vi "svc_Conditional Merge Array of Errors.vi"(7 "condition met":bool[](array[boolean]), 10 "possible errors and warnings":errorcluster[](array[cluster]), 11 "error in":errorcluster) -> (3 "error out":errorcluster)   [LabVIEW 2017]
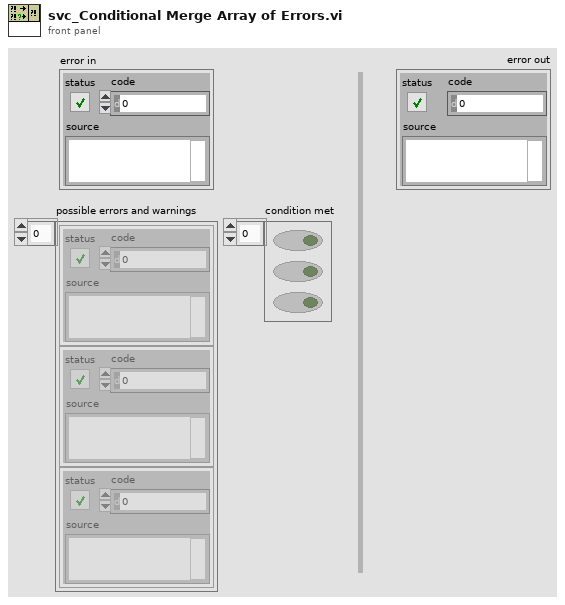
[diagram p1: front panel]
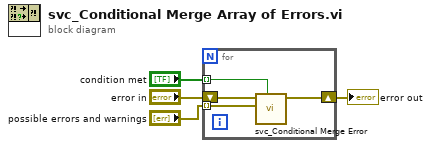
[diagram p0: block diagram]
diagram:
  n1 = for {
    shift-right: [w7] -> w4
    shift-left: "error in" -> [w8]
    tunnel: "possible errors and warnings" -> [w6] mode=indexing
    tunnel: "condition met" -> [w5] mode=indexing
    n2 = call <vilib>:"svc_Conditional Merge Error.vi"("merge"=w5, "new error"=w6, "error in (no error)"=w8) -> ("error out"=w7:errorcluster)  [unwired: 8 in]
  }
  "error out" <- w4
